vi "FunctDataMgr.Update Numeric Data.vi"(8 "error in (no error)":errorcluster, 10 "Data.Num":T1[](array[typedef]) {"Status" items=["LOG", "PASS", "FAIL", "ERROR"]}, 11 "FunctDataMgr in":refnum<class "FunctDataMgr.lvclass">) -> (0 "error out":errorcluster, 3 "FunctDataMgr out":refnum<class "FunctDataMgr.lvclass">)   [LabVIEW 2018, in "FunctDataMgr.lvclass"]
uses:
  FunctDataMgr.lvclass
  Results/Result.Numeric.ctl
  Results/Result.Limit Type.ctl
  Results/Result.Measurement and Attribute Item Status.ctl
  FunctDataMgr.lvclass/FunctDataMgr.ctl
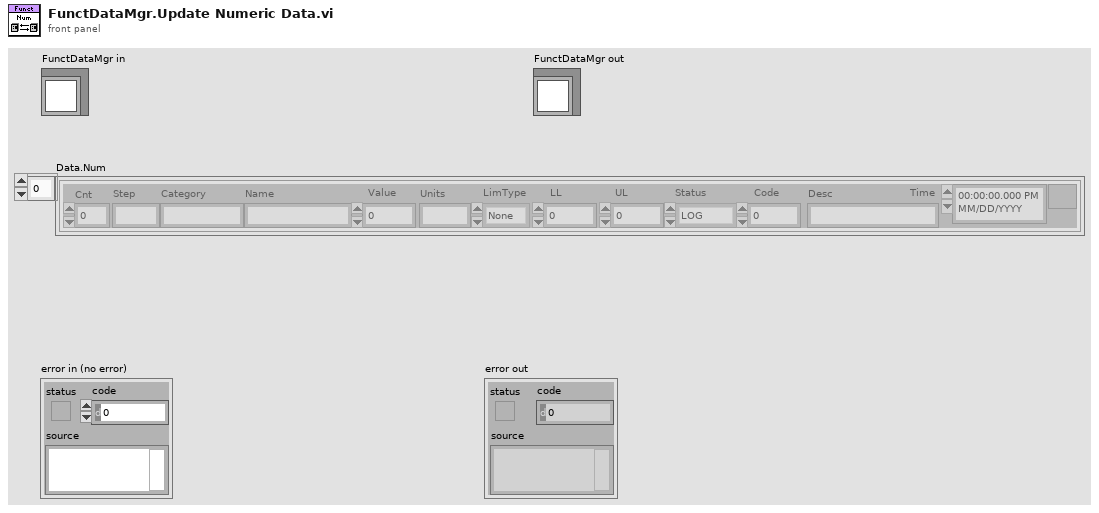
[diagram p1: front panel]
types:
  T1 = typedef "Result.Numeric.ctl" = cluster{"Cnt":i32, "Step":string, "Category":string, "Name":string, "Value":dbl, "Units":string, "LimType":T2, "LL":dbl, "UL":dbl, "Status":T3, "Code":i32, "Desc":string, "Time":timestamp}
  T2 = typedef "Result.Limit Type.ctl" = enum16{"None", "EQ", "NE", "GT", "LT", "GE", "LE", "GTLT", "GELE", "GELT", "GTLE", "LTGT", "LEGE", "LEGT", "LTGE", "Contains", "NotContains"}
  T3 = typedef "Result.Measurement and Attribute Item Status.ctl" = i32
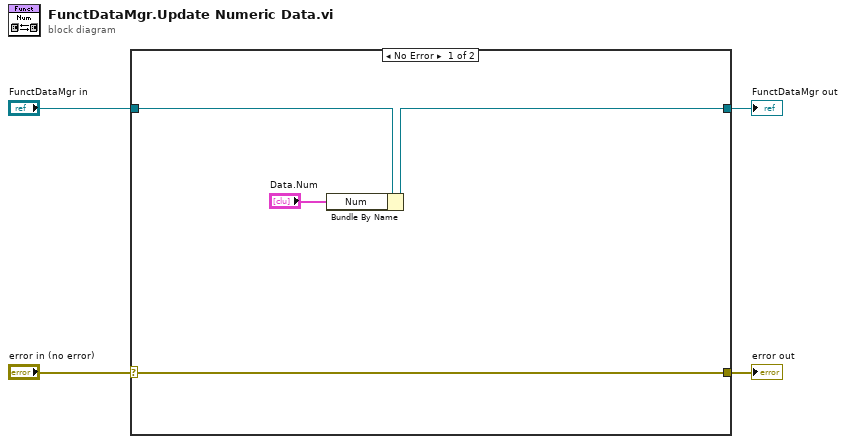
[diagram p0: block diagram]
diagram:
  n1 = case shown="No Error" "error in (no error)" {
    selector: "error in (no error)" -> [w8 w10]
    tunnel: [w8 w10] -> w3
    tunnel: [w6 w9] -> w1
    tunnel: "FunctDataMgr in" -> [w7 w9]
    frame No Error {
      n2 = Bundle By Name(cluster=w7, "Num"="Data.Num") -> (w6:refnum<class "FunctDataMgr.lvclass">)
    }
    frame Error {
    }
  }
  "error out" <- w3
  "FunctDataMgr out" <- w1
